vi "Configure Serial Port.vi"(5 "Timeout":u32=10000, 6 "Flow Control":u16(ring) items=["None", "XON/XOFF", "RTS/CTS", "XON/XOFF & RTS/CTS", "DTR/DSR", "XON/XOFF & DTR/DSR"], 7 "data bits":u16, 8 "error in (no error)":errorcluster, 9 "Parity":u16(ring)=2 items=["None", "Odd", "Even", "Mark", "Space"], 10 "Baud Rate":u32=9600, 11 "VISA Refnum in":refnum<visa-resource-name>) -> (0 "error out":errorcluster)   [LabVIEW 2021, in "Serial Shared Components.lvlib"]
doc: "Configures a selected serial port with various options."
uses:
  Serial Shared Components.lvlib
  <vilib>/Instr/_visa.llb/VISA Flush IO Buffer Mask.ctl
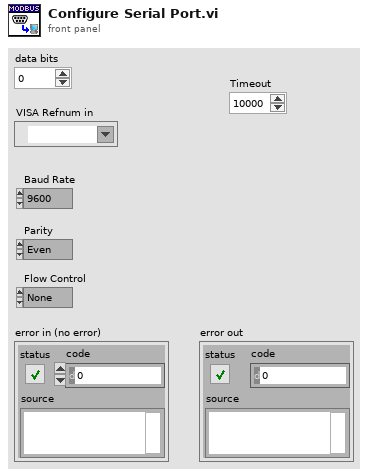
[diagram p1: front panel]
types:
  T1 = typedef "VISA Flush IO Buffer Mask.ctl" = u16
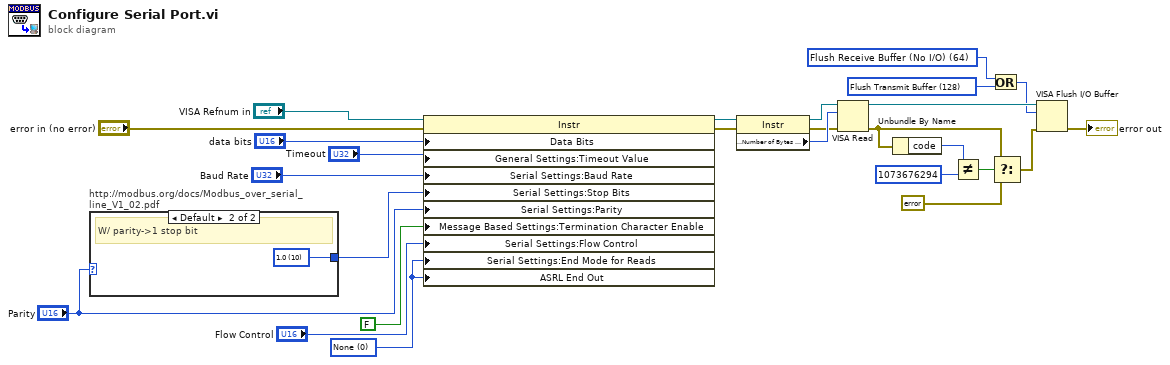
[diagram p0: block diagram]
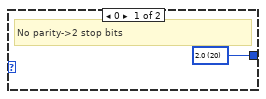
[diagram p2: hidden frame]
diagram:
  w15 = T1 128 items=["Flush Receive Buffer"=16, "Write Transmit Buffer to Device"=32, "Flush Receive Buffer (No I/O)"=64, "Flush Transmit Buffer"=128] ("Mask")
  w14 = T1 64 items=["Flush Receive Buffer"=16, "Write Transmit Buffer to Device"=32, "Flush Receive Buffer (No I/O)"=64, "Flush Transmit Buffer"=128] ("Mask")
  w8 = u16 0 items=["None", "LastBit", "TermChar"] ("Serial Settings:Serial End Mode for Reads")
  n1 = case "http://modbus.org/docs/Modbus_over_serial_line_V1_02.pdf" shown="Default" "Parity" {
    tunnel: [w27 w28] -> w12
    frame 0 {
      w27 = u16 20 items=["1.0"=10, "1.5"=15, "2.0"=20] ("Serial Settings:Serial Stop Bits")
      # "No parity->2 stop bits"
    }
    frame Default {
      w28 = u16 10 items=["1.0"=10, "1.5"=15, "2.0"=20] ("Serial Settings:Serial Stop Bits")
      # "W/ parity->1 stop bit"
    }
  }
  n2 = property class="Instr"(reference="VISA Refnum in", error in="error in (no error)", "Data Bits"="data bits", "General Settings:Timeout Value"="Timeout", "Serial Settings:Baud Rate"="Baud Rate", "Serial Settings:Stop Bits"=w12, "Serial Settings:Parity"="Parity", "Message Based Settings:Termination Character Enable"=FALSE, "Serial Settings:Flow Control"="Flow Control", "Serial Settings:End Mode for Reads"=w8, "ASRL End Out"=w8) -> (reference out=w20:refnum<visa-resource-name>, error out=w19:errorcluster)
  n3 = property class="Instr"(reference=w20, error in=w19) -> (reference out=w22:refnum<visa-resource-name>, error out=w9:errorcluster, "Serial Settings:Number of Bytes at Serial Port"=w23:u32)
  n4 = VISA Read(VISA resource name=w22, byte count=w23, error in (no error)=w9) -> (VISA resource name out=w21:refnum<visa-resource-name>, error out=w2:errorcluster)  [unwired: 2 out]
  n5 = Unbundle By Name(w2) -> ("code"=w7:i32)
  n6 = Not Equal?(x=w7, y=1073676294) -> (x != y?=w5:bool)
  n7 = Or(x=w14, y=w15) -> (x .or. y?=w13:T1)
  n8 = Select(t=w2, s=w5, f=errorcluster {"status"=FALSE, "code"=0, "source"=""}) -> (s? t:f=w1:errorcluster)
  n9 = VISA Flush I/O Buffer(VISA resource name=w21, mask (16)=w13, error in (no error)=w1) -> (error out=→"error out":errorcluster)  [unwired: 1 out]
